vi "Credit update.vi"(8 "error in (no error)":errorcluster, 10 "Creditp":dbl, 11 "UI Actor in":refnum<class "UI Actor.lvclass">) -> (0 "error out":errorcluster, 3 "UI Actor out":refnum<class "UI Actor.lvclass">)   [LabVIEW 2020, in "UI Actor.lvlib" / "UI Actor.lvclass"]
uses:
  UI Actor.lvclass
  UI Actor.lvclass/UI Actor.ctl
  MSG Messages/Update msg Msg/Update msg Msg.lvclass/Update msg Msg.ctl
  <vilib>/ActorFramework/Message Enqueuer/Message Enqueuer.lvclass/Message Enqueuer.ctl
  <vilib>/ActorFramework/Message Enqueuer/Enqueue.vi
  MSG Messages/Update msg Msg/Update msg Msg.lvclass
  C:/Program Files/National Instruments/LabVIEW 2020/vi.lib/ActorFramework/Message/Message.lvclass
  <vilib>/ActorFramework/Message Priority Queue/Priority Enqueue.vi
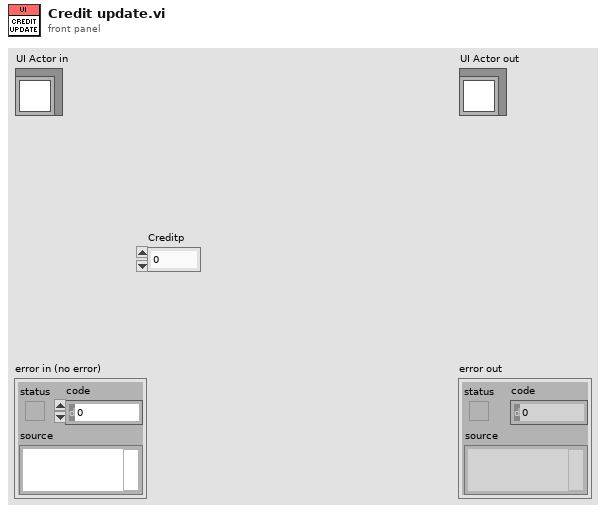
[diagram p1: front panel]
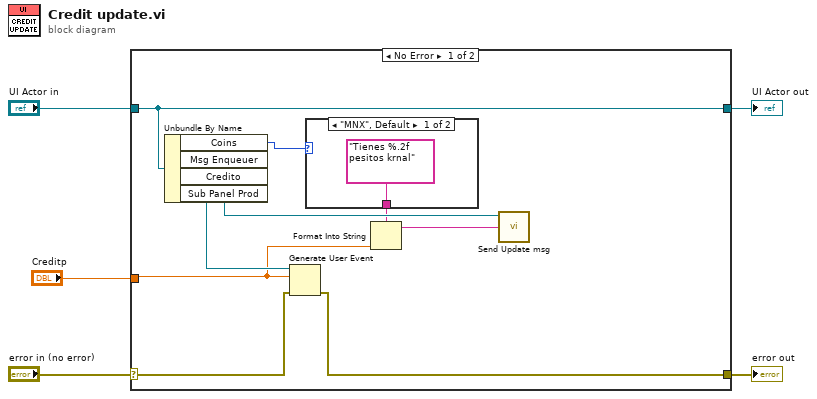
[diagram p0: block diagram]
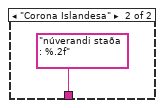
[diagram p2: hidden frame]
diagram:
  n1 = case shown="No Error" "error in (no error)" {
    selector: "error in (no error)" -> [w12 w18]
    tunnel: [w11 w18] -> w4
    tunnel: [w14 w17] -> w2
    tunnel: "UI Actor in" -> [w14 w17]
    tunnel: "Creditp" -> [w7 _]
    frame No Error {
      n2 = Unbundle By Name(w14) -> ("Coins"=w6:enum16{"MNX", "Corona Islandesa"}, "Msg Enqueuer"=w10:refnum<class "Message Enqueuer.lvclass">, "Credito"=w13:refnum<user-event>)  [unwired: 1 out]
      n3 = Generate User Event(user event=w13, event data cluster=w7, error in=w12) -> (error out=w11:errorcluster)  [unwired: 1 in, 1 out]
      n4 = case shown="\"MNX\", Default" w6 {
        tunnel: ["Tienes %.2f pesitos krnal" ("format string") "núverandi staða : %.2f" ("format string")] -> w8
        frame "MNX", Default {
        }
        frame "Corona Islandesa" {
        }
      }
      n5 = Format Into String(format string=w8, w7) -> (resulting string=w9:string)  [unwired: 2 in, 1 out]
      n6 = call "Send Update msg.vi"("Update msg"=w9, "Message Enqueuer"=w10) -> ()  [unwired: 8 in, 2 out]
    }
    frame Error {
    }
  }
  "error out" <- w4
  "UI Actor out" <- w2
